vi "Actor Core.vi"(8 "error in":errorcluster, 11 "Station Actor in":refnum<class "Station Actor.lvclass">) -> (0 "error out":errorcluster, 3 "Actor out":refnum<class "Actor.lvclass">)   [LabVIEW 2019, in "Station Actor.lvlib" / "Station Actor.lvclass"]
doc: "(<B>Filename</B>: Actor Framework.lvlib:Actor.lvclass:Actor Core.vi)\n\nReceives messages to the actor, reacts to them, and initiates any error handling that may shut the actor down.\n\nDescendant classes may override this VI to append parallel tasks for the actor to complete while it handles messages. Overrides use the Call Parent Method node."
uses:
  Station Actor.lvclass
  C:/Program Files (x86)/National Instruments/LabVIEW 2019/vi.lib/ActorFramework/Actor/Actor.lvclass
  <vilib>/ActorFramework/Actor/Actor.lvclass
  Custom Controls/Tester Rx Dataset.ctl
  Custom Controls/Tester Tx Dataset.ctl
  Station Actor.lvclass/Station Actor.ctl
  <vilib>/ActorFramework/Actor/Actor.lvclass/Actor.ctl
  <vilib>/ActorFramework/Message Enqueuer/Message Enqueuer.lvclass/Message Enqueuer.ctl
  PLC Sim Controller/PLC Sim Controller Actor Messages/Set PauseResume Msg/Set PauseResume Msg.lvclass/Set PauseResume Msg.ctl
  <vilib>/ActorFramework/Message Enqueuer/Init from Existing Queue.vi
  <vilib>/ActorFramework/Message Enqueuer/Enqueue.vi
  Station Actor Messages/Set Tester Tx Msg/Set Tester Tx Msg.lvclass
  C:/Program Files (x86)/National Instruments/LabVIEW 2019/vi.lib/ActorFramework/Message/Message.lvclass
  <vilib>/ActorFramework/Stop Msg/Stop Msg.lvclass
  PLC Sim Controller/PLC Sim Controller Actor Messages/Set PauseResume Msg/Set PauseResume Msg.lvclass
  Station Actor Messages/Set Tester Rx Msg/Set Tester Rx Msg.lvclass
  Station Actor Messages/Reset all components Msg/Reset all components Msg.lvclass
  <vilib>/ActorFramework/Message Priority Queue/Priority Enqueue.vi
  <vilib>/ActorFramework/Message Enqueuer/Message Enqueuer.lvclass
panel:
  in  "Auto":bool
  in  "Reset":bool
  in  "Run":bool
  out "Tester Tx":T1
  in  "Tester Rx":T2={"Start"=FALSE, "NestStatus"=FALSE, "PalletID"=0, "BarcodeData"="P:10-000001R:04S:QMC2200001", "StepEcho"=0, "Cylinder_1"=FALSE, "Cylinder_2"=FALSE, "Cylinder_3"=FALSE, "Cylinder_4"=FALSE, "Cylinder_5"=FALSE, "ResultsAck"=FALSE, "Reset"=FALSE, "Stop"=FALSE, "FaultCode"=0}
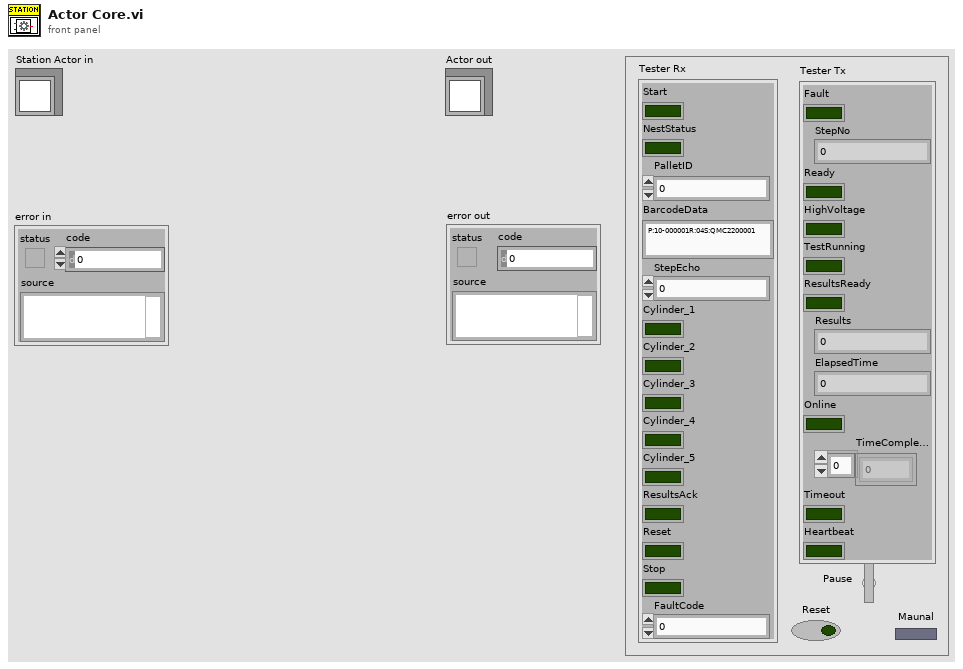
[diagram p1: front panel]
types:
  T1 = typedef "Station Actor.lvlib/Station Actor.lvclass/Tester Tx Dataset.ctl" = cluster{"Fault":bool, "StepNo":u32, "Ready":bool, "HighVoltage":bool, "TestRunning":bool, "ResultsReady":bool, "Results":u32, "ElapsedTime":u32, "Online":bool, "TimeCompleted":i32[], "Timeout":bool, "Heartbeat":bool}
  T2 = typedef "Station Actor.lvlib/Station Actor.lvclass/Tester Rx Dataset.ctl" = cluster{"Start":bool, "NestStatus":bool, "PalletID":u32, "BarcodeData":string, "StepEcho":u32, "Cylinder_1":bool, "Cylinder_2":bool, "Cylinder_3":bool, "Cylinder_4":bool, "Cylinder_5":bool, "ResultsAck":bool, "Reset":bool, "Stop":bool, "FaultCode":u32}
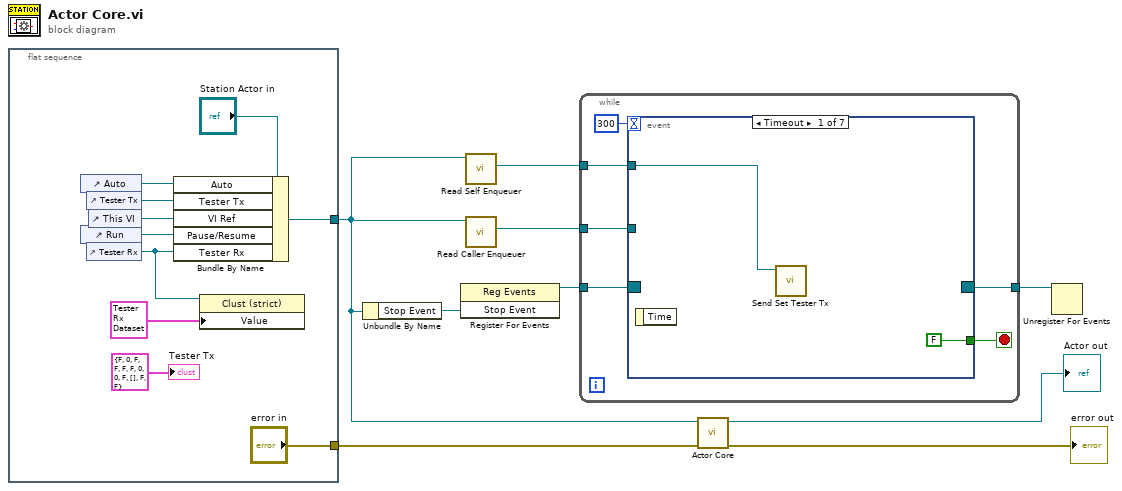
[diagram p0: block diagram]
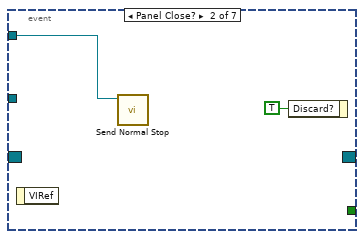
[diagram p2: hidden frame]
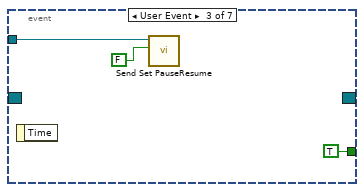
[diagram p3: hidden frame]
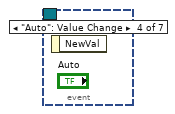
[diagram p4: hidden frame]
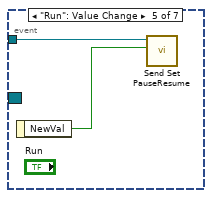
[diagram p5: hidden frame]
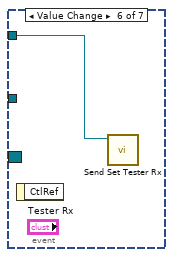
[diagram p6: hidden frame]
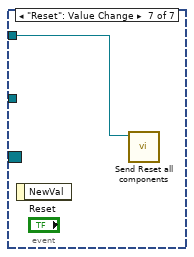
[diagram p7: hidden frame]
diagram:
  n1 = flat-sequence {
    tunnel: [w15] -> w2
    tunnel: ["error in"] -> w1
    frame #0 {
      n2 = control-ref of="Auto"() -> (w13:refnum<vi>)
      n3 = control-ref of="Run"() -> (w16:refnum<vi>)
      n4 = control-ref of="Tester Tx"() -> (w18:refnum<vi>)
      n5 = control-ref of="Tester Rx"() -> (w11:refnum<vi>)
      n6 = control-ref of="This VI"() -> (w17:refnum<vi>)
      n7 = Bundle By Name(cluster="Station Actor in", "Auto"=w13, "Tester Tx"=w18, "VI Ref"=w17, "Pause/Resume"=w16, "Tester Rx"=w11) -> (w15:refnum<class "Station Actor.lvclass">)
      n8 = property class="Clust (strict)"(reference=w11, "Value"=T2 {"Start"=FALSE, "NestStatus"=FALSE, "PalletID"=0, "BarcodeData"="P:10-000001R:04S:QMC2200001", "StepEcho"=0, "Cylinder_1"=FALSE, "Cylinder_2"=FALSE, "Cylinder_3"=FALSE, "Cylinder_4"=FALSE, "Cylinder_5"=FALSE, "ResultsAck"=FALSE, "Reset"=FALSE, "Stop"=FALSE, "FaultCode"=0}) -> ()  [unwired: 1 in, 2 out]
      "Tester Tx" <- T1 {"Fault"=FALSE, "StepNo"=0, "Ready"=FALSE, "HighVoltage"=FALSE, "TestRunning"=FALSE, "ResultsReady"=FALSE, "Results"=0, "ElapsedTime"=0, "Online"=FALSE, "TimeCompleted"=[], "Timeout"=FALSE, "Heartbeat"=FALSE} ("Tester Tx")
    }
  }
  n9 = Unbundle By Name(w2) -> ("Stop Event"=w7:refnum<user-event>)
  n10 = register-events ("Main Register for Events")(w7) -> (reference out=w4:refnum<event-registration>)  [unwired: 2 in, 1 out]
  n11 = call <vilib>:"Read Self Enqueuer.vi"("Actor"=w2) -> ("Self Enqueuer"=w6:refnum<class "Message Enqueuer.lvclass">)  [unwired: 10 in]
  n12 = call <vilib>:"Read Caller Enqueuer.vi"("Actor"=w2) -> ("Caller Enqueuer"=w5:refnum<class "Message Enqueuer.lvclass">)  [unwired: 10 in]
  n13 = while {
    tunnel: w6 -> [w24]
    tunnel: w5 -> [w23]
    tunnel: w4 -> [w22]
    tunnel: [w21] -> w3
    stop <- w25 stop-if-true
    n14 = event shown="[0] Timeout" {
      selector: w22 -> [_ _ _ _ _ _ _]
      dyn-events: [_ _ _ _ _ _ _] -> w21
      timeout: 300 -> [_ _ _ _ _ _ _]
      tunnel: [FALSE _ TRUE _ _ _ _] -> w25
      tunnel: w24 -> [w26 w28 _ _ _ w35 w36]
      tunnel: w23 -> [_ _ w30 _ w34 _ _]
      event Timeout {
        n15 = event-data() -> ()  [unwired: 1 in, 1 out]
        n16 = call "Send Set Tester Tx.vi"("Message Enqueuer"=w26) -> ()  [unwired: 9 in, 2 out]
      }
      event Panel Close? {
        n17 = event-data() -> ()  [unwired: 1 in, 1 out]
        n18 = call <vilib>:"Send Normal Stop.vi"("Message Enqueuer"=w28) -> ()  [unwired: 10 in, 1 out]
        n19 = event-data("Discard?"=TRUE) -> ()  [unwired: 1 in, 1 out]
      }
      event User Event {
        n20 = event-data() -> ()  [unwired: 1 in, 1 out]
        n21 = call "Send Set PauseResume.vi"("Pause/Resume"=FALSE, "Message Enqueuer"=w30) -> ()  [unwired: 8 in, 2 out]
      }
      event "Auto": Value Change {
        n22 = event-data() -> ()  [unwired: 1 in, 1 out]
      }
      event "Run": Value Change {
        n23 = event-data() -> ("NewVal"=w33:bool)  [unwired: 1 in]
        n24 = call "Send Set PauseResume.vi"("Pause/Resume"=w33, "Message Enqueuer"=w34) -> ()  [unwired: 8 in, 2 out]
      }
      event Value Change {
        n25 = event-data() -> ()  [unwired: 1 in, 1 out]
        n26 = call "Send Set Tester Rx.vi"("Message Enqueuer"=w35) -> ()  [unwired: 9 in, 2 out]
      }
      event "Reset": Value Change {
        n27 = event-data() -> ()  [unwired: 1 in, 1 out]
        n28 = call "Send Reset all components.vi"("Message Enqueuer"=w36) -> ()  [unwired: 9 in, 2 out]
      }
    }
  }
  n29 = call-parent "Actor Core.vi"("error in"=w1, "Actor in"=w2) -> ("error out"=→"error out":errorcluster, "Actor out"=→"Actor out":refnum<class "Actor.lvclass">)  [unwired: 8 in]
  n30 = Unregister For Events(event registration refnum=w3) -> ()  [unwired: 1 in, 1 out]
